vi "satellite simulator control.vi"() -> ()   [LabVIEW 2012]
uses:
  <vilib>/Utility/error.llb/DialogType.ctl
  <vilib>/DAQmx/create/channels.llb/DAQmx Create Channel (DO-Digital Output).vi
  <vilib>/Instr/_visa.llb/VISA Configure Serial Port (Instr).vi
  <vilib>/vision/NI_Vision_Development_Module.lvlib
  <vilib>/ptbypt/NI_PtbyPt.lvlib
panel:
  in  "Control Value":sgl=1.5 format="%.4f"
  in  "Control Mode":u16(ring) items=["Acceleration", "Speed", "Torque"]
  in  "Address":i32=11
  in  "Dst":i32=36
  in  "stop bits":u16(ring)=10 items=["1.0"=10, "1.5"=15, "2.0"=20]
  in  "VISA resource name (write) 2":refnum<visa-resource-name>="COM4"
  in  "flow control":u16(ring) items=["None"=0, "XON/XOFF"=1, "RTS/CTS"=2, "DTR/DSR"=4]
  in  "parity (0:none)":u16(ring) items=["None", "Odd", "Even", "Mark", "Space"]
  in  "data bits (8)":u16=8 min=5 max=8 step=1
  in  "baud rate (115200)":u32=115200
  out "bytes written":u32
  in  "bytes to read":u32=5
  out "read string":string
  out "bytes read":u32
  out "Filtered Ohmega":dbl format="%0.2f"
  in  "VISA resource name":refnum<visa-resource-name>
  out "read buffer":string
  out "Ohmega":dbl[](graph)
  out "Filtered Ohmega":dbl[](graph)
  in  "Floating":bool
  in  "Thruster 8":bool
  in  "Thruster 7":bool
  in  "Thruster 6":bool
  in  "Thruster 5":bool
  in  "Thruster 4":bool
  in  "Thruster 3":bool
  in  "Thruster 2":bool
  in  "Truster1":bool
  in  "Thrusters Bundled":bool=TRUE
  in  "Manual Control Mode (Default)":bool
  in  "Up":bool
  in  "Right":bool
  in  "Down":bool
  in  "Left":bool
  in  "Stop 2":bool
  in  "CntrClk":bool
  in  "ClkWise":bool
  in  "Angular Acceleration":u16(ring) items=["Fast", "Slow"]
  in  "Duty Cycle":dbl=1.0
  in  "Automatic PD Position Controller":bool
  in  "Pixel-Distance Ratio (pix/cm)":dbl=8.26
  in  "Remote Logger Status":bool
  in  "Downlink Object Data?":bool
  in  "Remote Port":u16=61557
  in  "Local Port":u16=61556
  in  "Remote Host":string="localhost"
  in  "broadcast":bool
  in  "Maintain Attitude":bool
  out "alpha":dbl
  out "Objects":T1(array[cluster]) {"Aspect Ratio" format="%.2f"; "Orientation" format="%.2f"; "Area" format="%.2f"; "Object Center"."Y" format="%.2f"; "Object Center"."X" format="%.2f"}
  in  "Y Center Correction":dbl
  in  "X Center Correction":dbl
  out "Offset Degree":dbl
  in  "Y Desired":dbl
  in  "X Desired":dbl
  out "Vx (cm/s)":dbl
  out "Vy (cm/s)":dbl
  in  "OK Button":bool
  in  "Air Floating Status":bool
  in  "Control Freq":u32=20
  in  "Alpha Desired":dbl
  in  "STOP":bool caption="stop (F)"
  out "Image Out":T2(plugin-control)
  out "alpha (deg)":dbl
  out "dx (cm)":dbl
  out "dy (cm)":dbl
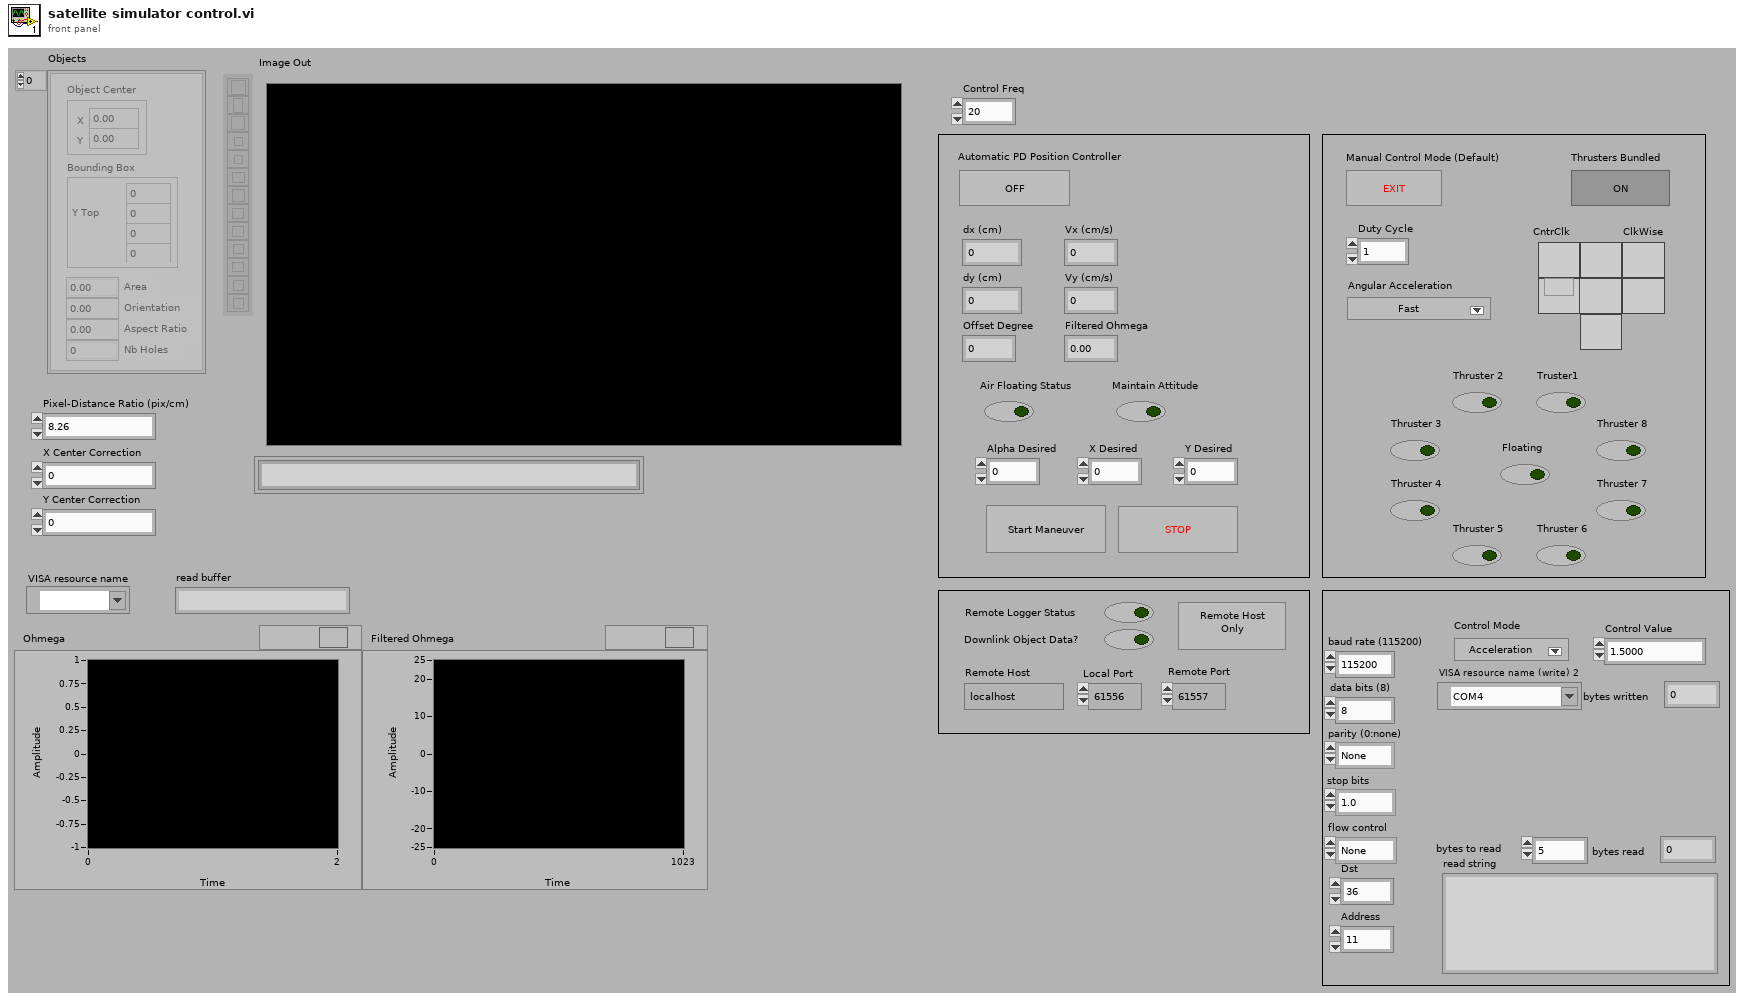
[diagram p1: front panel]
types:
  T1 = cluster{"Object Center":cluster{"X":sgl, "Y":sgl}, "Bounding Box":cluster{"X Left":i32, "Y Top":i32, "X Right":i32, "Y Bottom":i32}, "Area":sgl, "Orientation":sgl, "Aspect Ratio":sgl, "Nb Holes":i32}[]
  T2 = typedef "IMAQ Image.ctl" = refnum<image>
  T3 = typedef "DialogType.ctl" = u16
  T4 = cluster{"dx (cm)":dbl, "dy (cm)":dbl, "Offset Degree":dbl}
  T5 = cluster{"Objects":u16, "Threshold":i32, "Reject Border":bool, "Fill Holes":bool, "Min Object Size":bool, "Min Size":i32, "Max Object Size":bool, "Max Size":i32, "Show Search Area":bool, "Show Center":bool, "Show Bounding Box":bool}
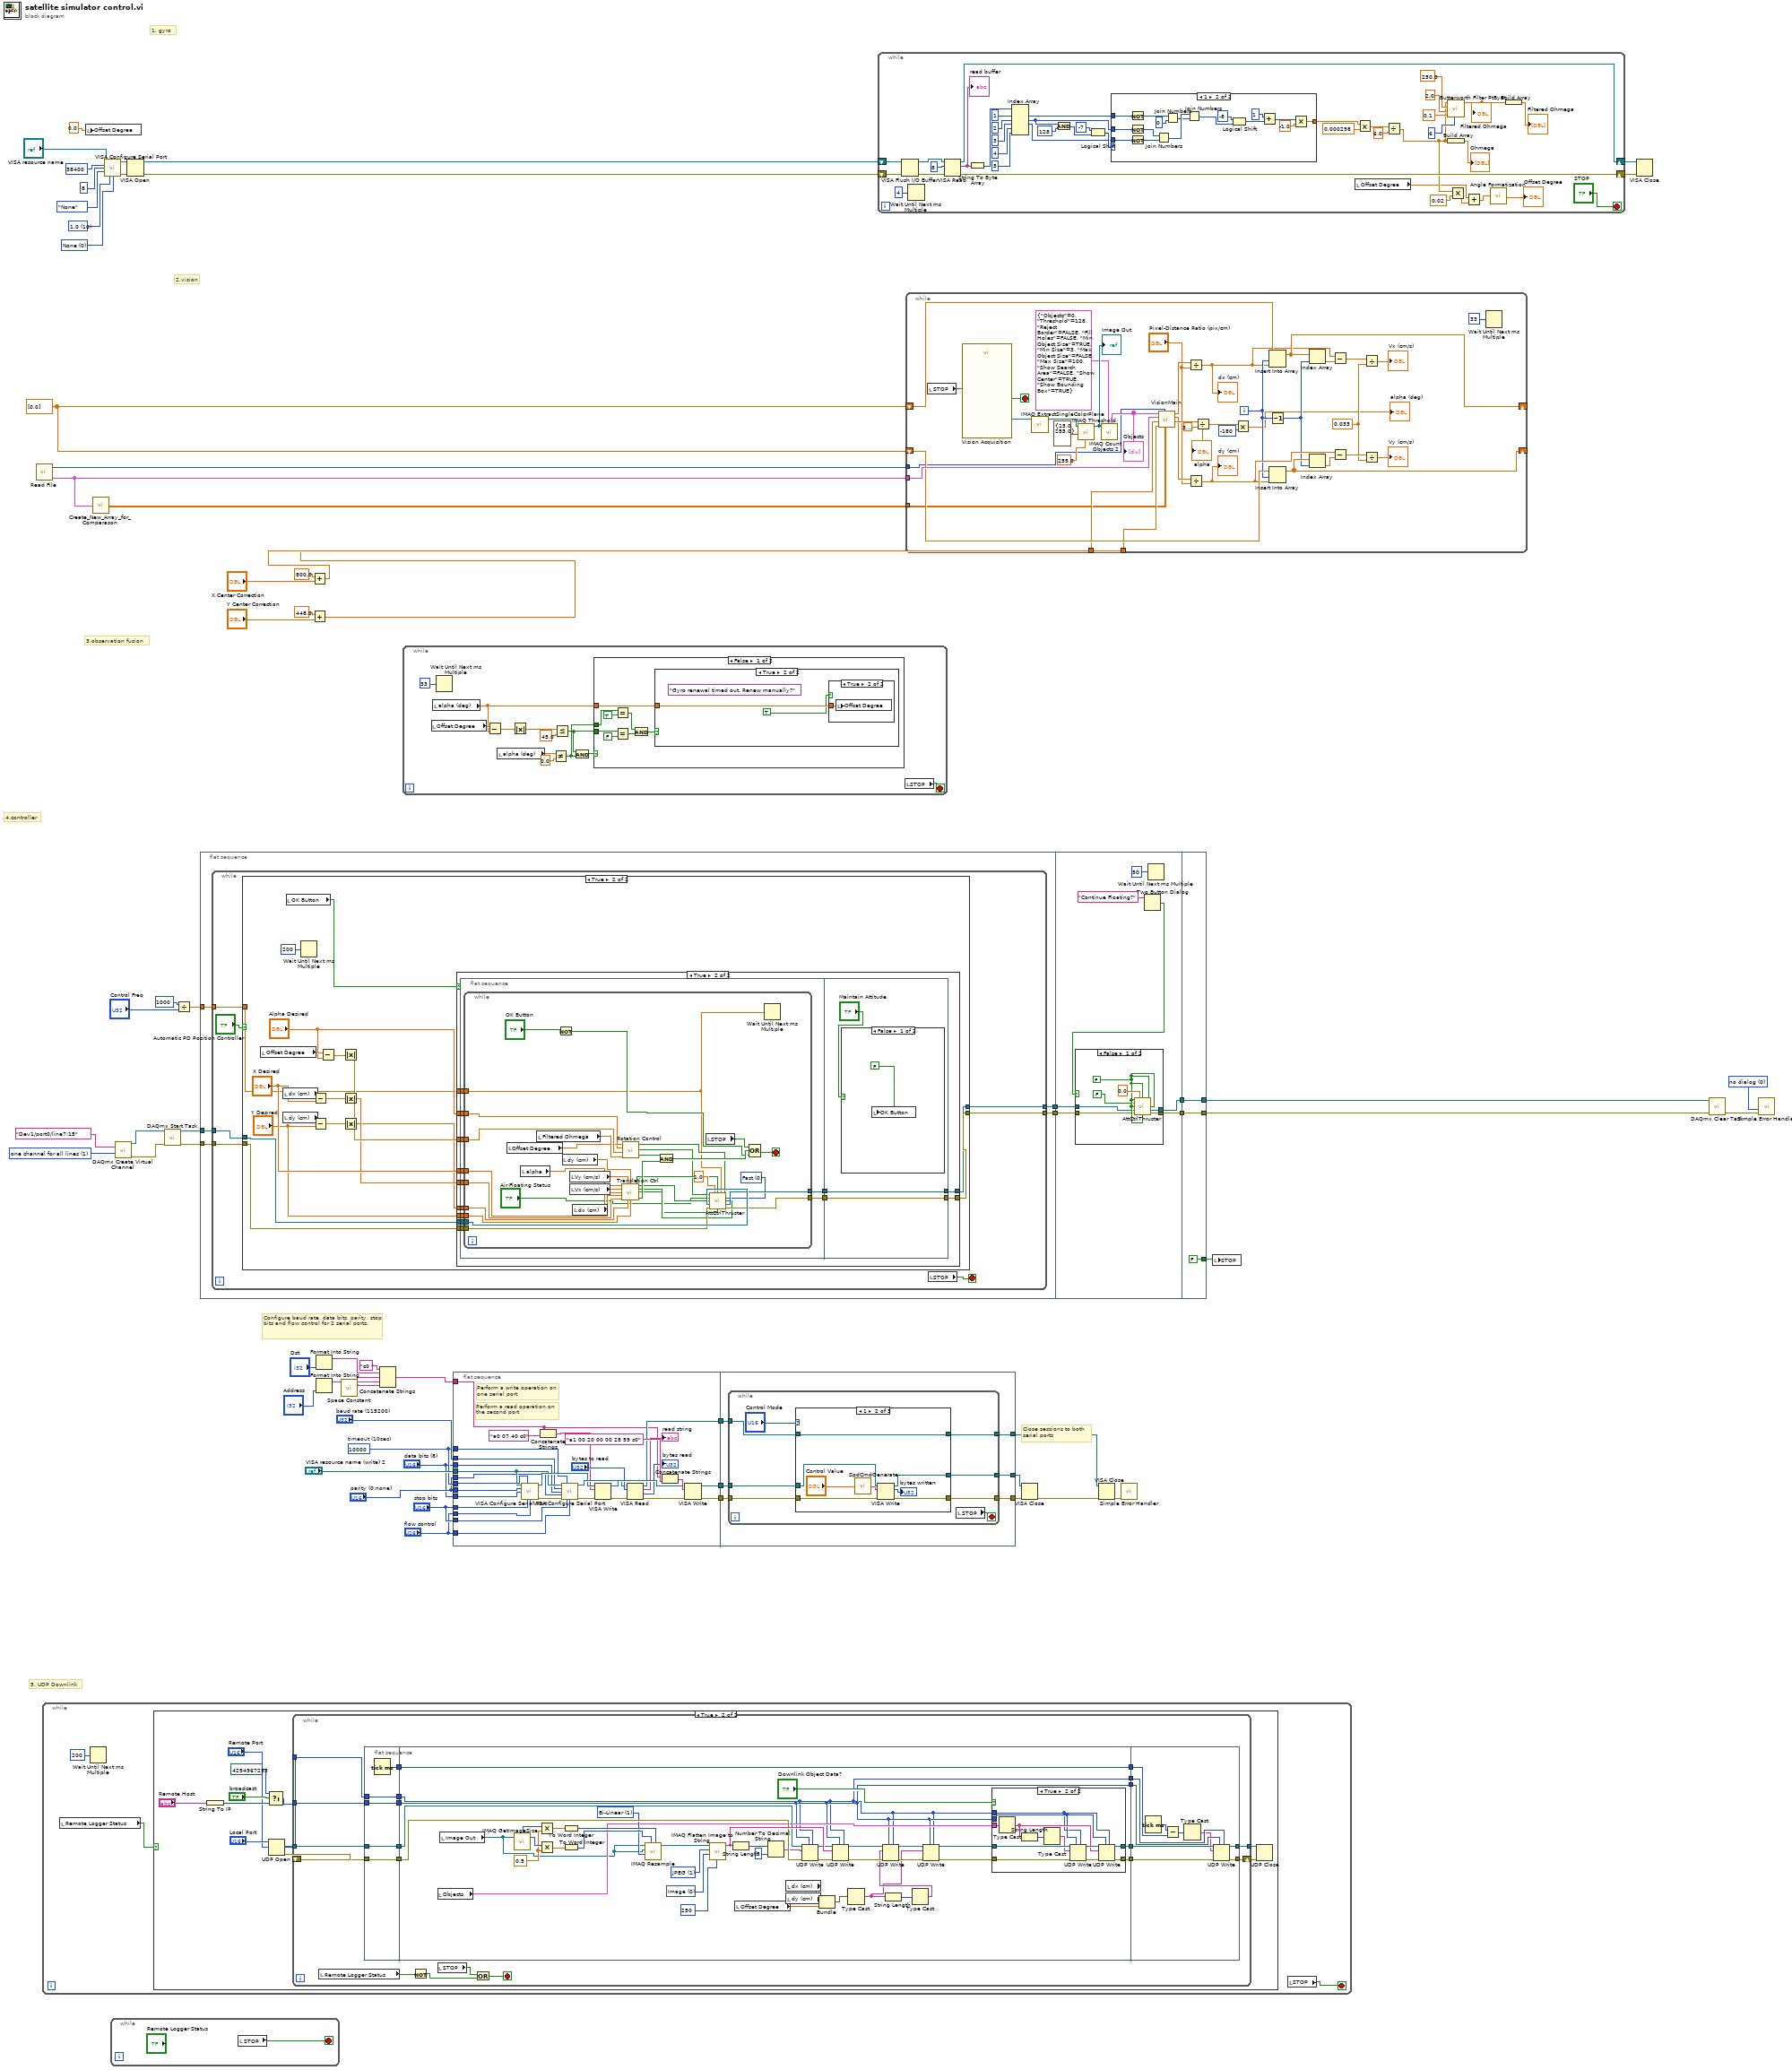
[diagram p0: block diagram]
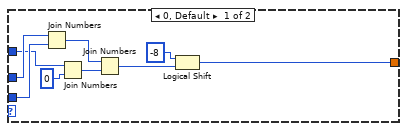
[diagram p4: hidden frame]
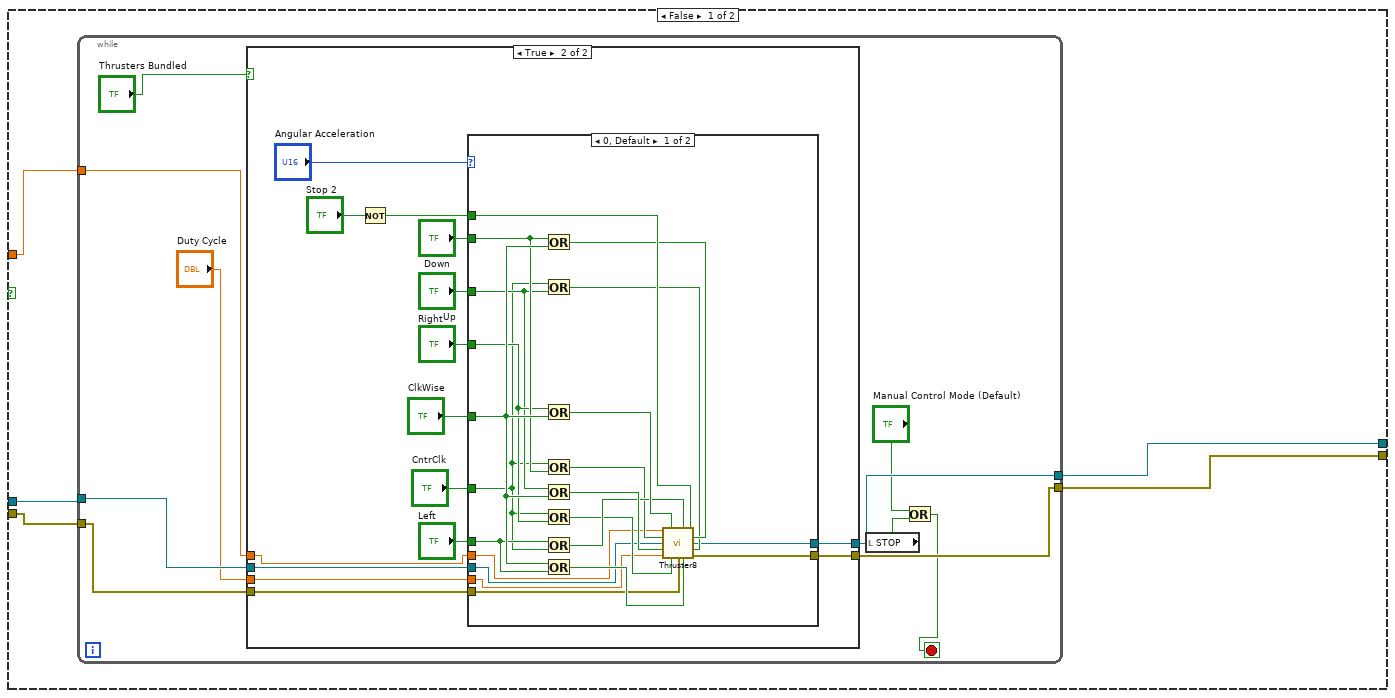
[diagram p7: hidden frame]
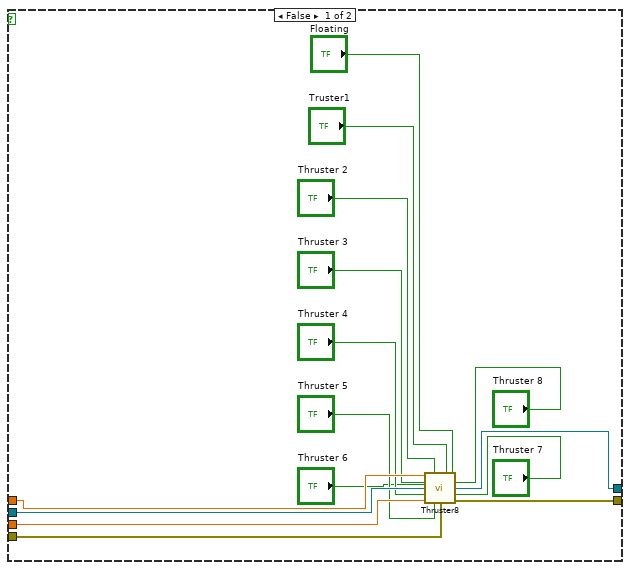
[diagram p8: hidden frame]
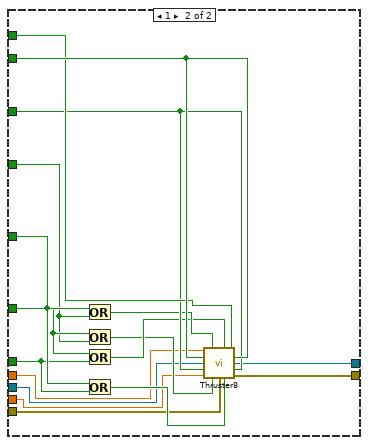
[diagram p9: hidden frame]
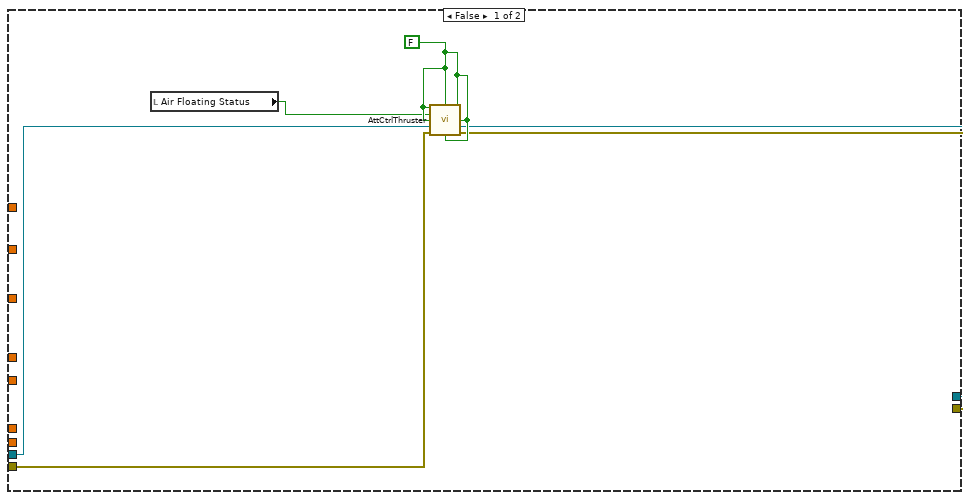
[diagram p10: hidden frame]
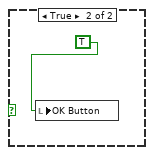
[diagram p11: hidden frame]
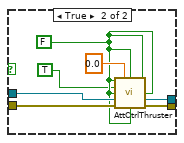
[diagram p12: hidden frame]
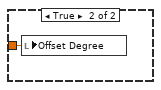
[diagram p15: hidden frame]
diagram:
  w6 = u32 10000  # timeout (10sec)
  w26 = u16 0 items=["None", "XON/XOFF", "RTS/CTS", "XON/XOFF & RTS/CTS", "DTR/DSR", "XON/XOFF & DTR/DSR"] ("flow control (0:none)")
  w28 = u16 10 items=["1.0"=10, "1.5"=15, "2.0"=20] ("stop bits (10: 1 bit)")
  w58 = T3 0 items=["no dialog", "OK message", "continue or stop message", "OK message + warnings", "continue/stop + warnings"] ("type of dialog (OK msg:1)")
  w61 = 1 items=["one channel for each line", "one channel for all lines"] ("line grouping")
  w47 = dbl[] [0.0]
  # "Close sessions to both serial ports"
  # "Configure baud rate, data bits, parity, stop bits and flow control for 2 serial ports."
  # "5. UDP Downlink"
  # "4.controller"
  # "3.observation fusion"
  # "2.vision"
  # "1. gyro"
  n1 = call "Read File.vi"() -> ("Objects"=w25:T1, "Total Obj"=w23:i32)  [unwired: 1 in]
  n2 = while {
    stop <- w65 stop-if-true
    n3 = local read "Remote Logger Status"() -> (w66:bool)
    n4 = Wait Until Next ms Multiple(millisecond multiple=u32 200) -> ()  [unwired: 1 out]
    n5 = case shown="True" w66 {
      frame False {
      }
      frame True {
        n6 = String To IP(1:"Remote Host") -> (0:w74:u32)
        n7 = Select(t=u32 4294967295, s="broadcast", f=w74) -> (s? t:f=w71:u32)
        n8 = UDP Open(11:"Local Port") -> (port=w70:refnum<k16>, 0:w69:errorcluster)  [unwired: 1 in, 4 out]
        n9 = while {
          tunnel: "Remote Port" -> [w97]
          tunnel: w71 -> [w96]
          tunnel: w70 -> [w95]
          tunnel: [w93] -> w68
          shift-right: [w92] -> w67
          shift-left: w69 -> [w94]
          stop <- w81 stop-if-true
          n10 = local read "Remote Logger Status"() -> (w79:bool)
          n11 = flat-sequence {
            tunnel: w95 -> [w99]
            tunnel: w97 -> [w100]
            tunnel: w96 -> [w101]
            tunnel: w94 -> [w102]
            tunnel: [w102] -> w91
            tunnel: [w101] -> w90
            tunnel: [w100] -> w89
            tunnel: [w99] -> w88
            tunnel: [w98] -> w87
            tunnel: [w122] -> w86
            tunnel: [w121] -> w85
            tunnel: w91 -> [w140]
            tunnel: w90 -> [w104]
            tunnel: w89 -> [w103]
            tunnel: w88 -> [w124]
            tunnel: [w123] -> w84
            tunnel: w87 -> [w123]
            tunnel: [w103] -> w83
            tunnel: [w104] -> w82
            tunnel: [w164] -> w93
            tunnel: [w158] -> w92
            tunnel: w86 -> [w159]
            tunnel: w85 -> [w165]
            tunnel: w84 -> [w166]
            tunnel: w83 -> [w163]
            tunnel: w82 -> [w162]
            frame #0 {
              n12 = Tick Count (ms)() -> (millisecond timer value=w98:u32)
            }
            frame #1 {
              w128 = u32 1 items=["Zero Order", "Bi-Linear", "Quadratic", "Cubic Spline"] ("Interpolation Type")
              w129 = 0.5
              w137 = 0 items=["Image", "Image and Vision Info", "Reference to Image"] ("Type of Flatten (Image and Vision Info)")
              w142 = 1 items=["None", "JPEG", "PACKED BINARY"] ("Compression (None)")
              n13 = local read "Objects"() -> (w119:T1)
              n14 = local read "Image Out"() -> (w118:T2)
              n15 = call "IMAQ GetImageSize"("Image"=w118) -> ("Y Resolution"=w130:i32, "X Resolution"=w131:i32)  [unwired: 3 in, 1 out]
              n16 = Multiply(x=w131, y=w129) -> (x*y=w133:dbl)
              n17 = Multiply(x=w130, y=w129) -> (x*y=w135:dbl)
              n18 = To Word Integer(number=w133) -> (16bit integer=w132:i16)
              n19 = To Word Integer(number=w135) -> (16bit integer=w134:i16)
              n20 = call "IMAQ Resample"("X Resolution"=w132, "Y Resolution"=w134, "Interpolation Type"=w128, "Image Dst"=w118, "Image Src"=w118) -> ("Image Dst Out"=w136:T2)  [unwired: 5 in, 1 out]
              n21 = call "IMAQ Flatten Image to String"("Quality (750)"=250, "Type of Flatten (Image and Vision Info)"=w137, "Compression (None)"=w142, "Image"=w136) -> ("Data String"=w141:string)  [unwired: 6 in, 1 out]
              n22 = String Length(string=w141) -> (length=w127:i32)
              n23 = local read "Offset Degree"() -> (w115:dbl)
              n24 = Number To Decimal String(number=w127, width (-)=i16 5) -> (decimal integer string=w126:string)
              n25 = local read "dx (cm)"() -> (w117:dbl)
              n26 = local read "dy (cm)"() -> (w116:dbl)
              n27 = UDP Write(address=w104, port or service name=w103, connection ID=w124, data in=w126, 8:w140) -> (error out=w139:errorcluster, 3:w138:refnum<k16>)  [unwired: 1 out]
              n28 = Bundle("dx (cm)"=w117, "dy (cm)"=w116, "Offset Degree"=w115) -> (w114:T4)  [unwired: 1 in]
              n29 = UDP Write(address=w104, port or service name=w103, connection ID=w138, data in=w141, 8:w139) -> (error out=w112:errorcluster, 3:w113:refnum<k16>)  [unwired: 1 out]
              n30 = Type Cast(x=w114) -> (*(type *) &x=w105:string)  [unwired: 1 in]
              n31 = String Length(string=w105) -> (length=w107:i32)
              n32 = Type Cast(x=w107) -> (*(type *) &x=w106:string)  [unwired: 1 in]
              n33 = UDP Write(address=w104, port or service name=w103, connection ID=w113, data in=w106, 8:w112) -> (error out=w111:errorcluster, 3:w109:refnum<k16>)  [unwired: 1 out]
              n34 = UDP Write(address=w104, port or service name=w103, connection ID=w109, data in=w105, 8:w111) -> (error out=w110:errorcluster, 3:w108:refnum<k16>)  [unwired: 1 out]
              n35 = case shown="True" "Downlink Object Data?" {
                tunnel: w119 -> [_ w157]
                tunnel: w110 -> [w145 w155]
                tunnel: [w145 w153] -> w122
                tunnel: w108 -> [w144 w152]
                tunnel: [w144 w150] -> w121
                tunnel: w104 -> [_ w147]
                tunnel: w103 -> [_ w146]
                frame False {
                }
                frame True {
                  n36 = Type Cast(x=w157) -> (*(type *) &x=w148:string)  [unwired: 1 in]
                  n37 = String Length(string=w148) -> (length=w156:i32)
                  n38 = Type Cast(x=w156) -> (*(type *) &x=w149:string)  [unwired: 1 in]
                  n39 = UDP Write(address=w147, port or service name=w146, connection ID=w152, data in=w149, 8:w155) -> (error out=w154:errorcluster, 3:w151:refnum<k16>)  [unwired: 1 out]
                  n40 = UDP Write(address=w147, port or service name=w146, connection ID=w151, data in=w148, 8:w154) -> (error out=w153:errorcluster, 3:w150:refnum<k16>)  [unwired: 1 out]
                }
              }
            }
            frame #2 {
              n41 = Tick Count (ms)() -> (millisecond timer value=w167:u32)
              n42 = Subtract(x=w167, y=w166) -> (x-y=w161:u32)
              n43 = Type Cast(x=w161) -> (*(type *) &x=w160:string)  [unwired: 1 in]
              n44 = UDP Write(address=w162, port or service name=w163, connection ID=w165, data in=w160, 8:w159) -> (error out=w158:errorcluster, 3:w164:refnum<k16>)  [unwired: 1 out]
            }
          }
          n45 = Not(x=w79) -> (.not. x?=w78:bool)
          n46 = local read "STOP"() -> (w80:bool)
          n47 = Or(x=w80, y=w78) -> (x .or. y?=w81:bool)
        }
        n48 = UDP Close(connection ID=w68, 8:w67) -> ()  [unwired: 2 out]
      }
    }
    n49 = local read "STOP"() -> (w65:bool)
  }
  n50 = local write "Offset Degree"(0.0 ("y")) -> ()
  n51 = call "Create_New_Array_for_Comparason.vi"("Captured Plots"=w25) -> ("Generated Distance Array"=w24:dbl[][])
  n52 = call-poly "VISA Configure Serial Port"("VISA resource name"="VISA resource name", "baud rate (9600)"=u32 38400, "data bits (8)"=u16 8, "parity (0:none)"=enum16{"None", "Odd", "Even", "Mark", "Space"}."None", "stop bits (10: 1 bit)"=w28, "flow control (0:none)"=w26) -> ("VISA resource name out"=w35:refnum<visa-resource-name>, "error out"=w34:errorcluster)  [unwired: 8 in]
  n53 = while {
    stop <- w168 stop-if-true
    n54 = local read "STOP"() -> (w168:bool)
  }
  n55 = call-poly <vilib>:"DAQmx Create Virtual Channel.vi"("lines"=tag "Dev1/port0/line7:15" ("Lines"), "line grouping"=w61) -> ("task out"=w59:refnum<k21>, "error out"=w60:errorcluster)  [unwired: 12 in]
  n56 = VISA Open(error in (no error)=w34, VISA resource name=w35) -> (VISA resource name=w33:refnum<visa-resource-name>, error out=w32:errorcluster)  [unwired: 3 in]
  n57 = call <vilib>:"DAQmx Start Task.vi"("task/channels in"=w59, "error in"=w60) -> ("task out"=w54:refnum<k21>, "error out"=w53:errorcluster)  [unwired: 12 in]
  n58 = Divide(x=u32 1000 ("milliseconds to wait"), y="Control Freq") -> (x/y=w50:dbl)
  n59 = flat-sequence {
    tunnel: w54 -> [w173]
    tunnel: w53 -> [w172]
    tunnel: w50 -> [w169]
    tunnel: [w171] -> w49
    tunnel: [w170] -> w48
    tunnel: w49 -> [w358]
    tunnel: w48 -> [w356]
    tunnel: [w357] -> w40
    tunnel: [w355] -> w39
    tunnel: [w374] -> w51
    tunnel: [w375] -> w52
    tunnel: w40 -> [w375]
    tunnel: w39 -> [w374]
    tunnel: [FALSE] -> w38
    frame #0 {
      n60 = while {
        tunnel: w173 -> [w180]
        tunnel: w172 -> [w179]
        tunnel: [w178] -> w171
        tunnel: [w177] -> w170
        tunnel: w169 -> [w175]
        stop <- w176 stop-if-true
        n61 = case shown="True" "Automatic PD Position Controller" {
          tunnel: w180 -> [w184 w282]
          tunnel: w179 -> [w183 w281]
          tunnel: [w181 w280] -> w178
          tunnel: [w182 w279] -> w177
          tunnel: w175 -> [w185 w265]
          frame False {
            n62 = while {
              tunnel: w185 -> [w195]
              tunnel: w184 -> [w194]
              tunnel: [w193] -> w182
              tunnel: [w192] -> w181
              tunnel: w183 -> [w191]
              stop <- w188 stop-if-true
              n63 = case shown="True" "Thrusters Bundled" {
                tunnel: w195 -> [w206 w218]
                tunnel: w194 -> [w210 w217]
                tunnel: [w207 w216] -> w193
                tunnel: [w208 w215] -> w192
                tunnel: w191 -> [w209 w214]
                tunnel: "Duty Cycle" -> [w205 w211]
                frame False {
                  n64 = call "Thruster8.vi"("period"=w206, "Thruster 2"="Thruster 2", "Truster1"="Truster1", "Floating"="Floating", "Thruster 3"="Thruster 3", "Thruster 8"="Thruster 8", "task in"=w210, "Thruster 4"="Thruster 4", "Thruster 7"="Thruster 7", "Duty Cycle"=w205, "Thruster 5"="Thruster 5", "error in"=w209, "Thruster 6"="Thruster 6") -> ("task out"=w207:refnum<k21>, "error out"=w208:errorcluster)  [unwired: 1 in]
                }
                frame True {
                  n65 = Not(x="Stop 2") -> (.not. x?=w212:bool)
                  n66 = case shown="0, Default" "Angular Acceleration" {
                    tunnel: w212 -> [w246 w262]
                    tunnel: "Down" -> [w238 w263]
                    tunnel: "Left" -> [w240 w256]
                    tunnel: "Up" -> [w234 w261]
                    tunnel: "Right" -> [w236 w254]
                    tunnel: "ClkWise" -> [w242 w260]
                    tunnel: "CntrClk" -> [w233 w257]
                    tunnel: w211 -> [w231 w252]
                    tunnel: w218 -> [w230 w251]
                    tunnel: w217 -> [w229 w247]
                    tunnel: [w228 w248] -> w216
                    tunnel: [w227 w249] -> w215
                    tunnel: w214 -> [w226 w250]
                    frame 0, Default {
                      n67 = Or(x=w238, y=w242) -> (x .or. y?=w241:bool)
                      n68 = Or(x=w233, y=w234) -> (x .or. y?=w232:bool)
                      n69 = Or(x=w236, y=w242) -> (x .or. y?=w244:bool)
                      n70 = Or(x=w233, y=w238) -> (x .or. y?=w237:bool)
                      n71 = Or(x=w234, y=w242) -> (x .or. y?=w245:bool)
                      n72 = Or(x=w233, y=w236) -> (x .or. y?=w235:bool)
                      n73 = Or(x=w240, y=w233) -> (x .or. y?=w239:bool)
                      n74 = Or(x=w242, y=w240) -> (x .or. y?=w243:bool)
                      n75 = call "Thruster8.vi"("period"=w230, "Thruster 2"=w244, "Truster1"=w239, "Floating"=w246, "Thruster 3"=w237, "Thruster 8"=w241, "task in"=w229, "Thruster 4"=w245, "Thruster 7"=w232, "Duty Cycle"=w231, "Thruster 5"=w235, "error in"=w226, "Thruster 6"=w243) -> ("task out"=w228:refnum<k21>, "error out"=w227:errorcluster)  [unwired: 1 in]
                    }
                    frame 1 {
                      n76 = Or(x=w260, y=w254) -> (x .or. y?=w259:bool)
                      n77 = Or(x=w257, y=w254) -> (x .or. y?=w253:bool)
                      n78 = Or(x=w257, y=w256) -> (x .or. y?=w255:bool)
                      n79 = Or(x=w260, y=w256) -> (x .or. y?=w258:bool)
                      n80 = call "Thruster8.vi"("period"=w251, "Thruster 2"=w259, "Truster1"=w255, "Floating"=w262, "Thruster 3"=w263, "Thruster 8"=w263, "task in"=w247, "Thruster 4"=w261, "Thruster 7"=w261, "Duty Cycle"=w252, "Thruster 5"=w253, "error in"=w250, "Thruster 6"=w258) -> ("task out"=w248:refnum<k21>, "error out"=w249:errorcluster)  [unwired: 1 in]
                    }
                  }
                }
              }
              n81 = local read "STOP"() -> (w190:bool)
              n82 = Or(x="Manual Control Mode (Default)", y=w190) -> (x .or. y?=w188:bool)
            }
          }
          frame True {
            n83 = local read "Offset Degree"() -> (w278:dbl)
            n84 = local read "dx (cm)"() -> (w274:dbl)
            n85 = local read "dy (cm)"() -> (w270:dbl)
            n86 = local read "OK Button"() -> (w266:bool)
            n87 = Wait Until Next ms Multiple(millisecond multiple=u32 200) -> ()  [unwired: 1 out]
            n88 = Subtract(x=w274, y="X Desired") -> (x-y=w272:dbl)
            n89 = Subtract(x=w270, y="Y Desired") -> (x-y=w268:dbl)
            n90 = Subtract(x=w278, y="Alpha Desired") -> (x-y=w276:dbl)
            n91 = Absolute Value(x=w276) -> (abs(x)=w275:dbl)
            n92 = Absolute Value(x=w272) -> (abs(x)=w271:dbl)
            n93 = Absolute Value(x=w268) -> (abs(x)=w267:dbl)
            n94 = case shown="True" w266 {
              tunnel: w282 -> [w286 w301]
              tunnel: w281 -> [w285 w300]
              tunnel: [w284 w299] -> w280
              tunnel: [w283 w298] -> w279
              tunnel: w265 -> [_ w297]
              tunnel: "Alpha Desired" -> [_ w296]
              tunnel: w275 -> [_ w295]
              tunnel: "X Desired" -> [_ w294]
              tunnel: w271 -> [_ w293]
              tunnel: "Y Desired" -> [_ w292]
              tunnel: w267 -> [_ w291]
              frame False {
                w288 = FALSE
                n95 = local read "Air Floating Status"() -> (w287:bool)
                n96 = call "AttCtrlThruster.vi"("ctclk"=w288, "Up"=w288, "clkwis"=w288, "Float"=w287, "Left"=w288, "Right"=w288, "task in"=w286, "error in"=w285, "Down"=w288) -> ("task out"=w283:refnum<k21>, "error out"=w284:errorcluster)  [unwired: 5 in]
              }
              frame True {
                n97 = flat-sequence {
                  tunnel: w301 -> [w312]
                  tunnel: w300 -> [w311]
                  tunnel: w297 -> [w308]
                  tunnel: w296 -> [w307]
                  tunnel: w295 -> [w306]
                  tunnel: w294 -> [w305]
                  tunnel: w293 -> [w304]
                  tunnel: w292 -> [w303]
                  tunnel: w291 -> [w302]
                  tunnel: [w310] -> w290
                  tunnel: [w309] -> w289
                  tunnel: [w348] -> w298
                  tunnel: [w349] -> w299
                  tunnel: w290 -> [w349]
                  tunnel: w289 -> [w348]
                  frame #0 {
                    n98 = while {
                      tunnel: w312 -> [w346]
                      tunnel: w311 -> [w345]
                      tunnel: [w343] -> w310
                      tunnel: [w344] -> w309
                      tunnel: w308 -> [w314]
                      tunnel: w307 -> [w324]
                      tunnel: w306 -> [w339]
                      tunnel: w305 -> [w323]
                      tunnel: w304 -> [w334]
                      tunnel: w303 -> [w322]
                      tunnel: w302 -> [w321]
                      stop <- w340 stop-if-true
                      w330 = u16 0 items=["Fast", "Slow"] ("Angular Acceleration")
                      n99 = local read "Offset Degree"() -> (w337:dbl)
                      n100 = local read "alpha"() -> (w318:dbl)
                      n101 = local read "Filtered Ohmega"() -> (w338:dbl)
                      n102 = Not(x="OK Button") -> (.not. x?=w319:bool)
                      n103 = local read "dy (cm)"() -> (w332:dbl)
                      n104 = local read "Vy (cm/s)"() -> (w333:dbl)
                      n105 = local read "Vx (cm/s)"() -> (w336:dbl)
                      n106 = local read "dx (cm)"() -> (w335:dbl)
                      n107 = call "Translation Ctrl.vi"("Alpha"=w318, "Filtered Speed Y"=w333, "Y In"=w332, "Filtered Speed X"=w336, "X In"=w335, "X Desired"=w323, "Original Difference X"=w334, "Original Difference Y"=w321, "Y Desired"=w322) -> ("Left"=w328:bool, "Right"=w327:bool, "Down"=w326:bool, "Up"=w325:bool, "Maneuver Complete?"=w329:bool)  [unwired: 2 in]
                      n108 = call "Rotation Control.vi"("Filtered Ohmega"=w338, "Original Difference"=w339, "Alpha Desired"=w324, "Alpha In"=w337) -> ("Maneuver Complete?"=w317:bool, "Counter-ClkWise Rot Ctrl"=w316:bool, "Clockwise Rot Ctrl"=w315:bool)
                      n109 = And(x=w317, y=w329) -> (x .and. y?=w331:bool)
                      n110 = local read "STOP"() -> (w341:bool)
                      n111 = call "AttCtrlThruster.vi"("ctclk"=w316, "Duty Cycle"=1.0, "Up"=w325, "Period"=w314, "clkwis"=w315, "Float"="Air Floating Status", "Angular Acceleration"=w330, "Left"=w328, "Right"=w327, "task in"=w346, "error in"=w345, "Down"=w326) -> ("task out"=w344:refnum<k21>, "error out"=w343:errorcluster)  [unwired: 2 in]
                      n112 = Compound Arithmetic op=OR(w341, w331, w319) -> (w340:bool)
                      n113 = Wait Until Next ms Multiple(millisecond multiple=w314) -> ()  [unwired: 1 out]
                    }
                  }
                  frame #1 {
                    n114 = case shown="False" "Maintain Attitude" {
                      frame False {
                        n115 = local write "OK Button"(FALSE) -> ()
                      }
                      frame True {
                        n116 = local write "OK Button"(TRUE) -> ()
                      }
                    }
                  }
                }
              }
            }
          }
        }
        n117 = local read "STOP"() -> (w176:bool)
      }
    }
    frame #1 {
      n118 = Two Button Dialog(message="Continue Floating?") -> (T button?=w352:bool)  [unwired: 2 in]
      n119 = case shown="False" w352 {
        tunnel: w358 -> [w361 w372]
        tunnel: [w359 w371] -> w357
        tunnel: w356 -> [w362 w370]
        tunnel: [w360 w369] -> w355
        frame False {
          w364 = FALSE
          n120 = call "AttCtrlThruster.vi"("ctclk"=w364, "Duty Cycle"=0.0, "Up"=w364, "clkwis"=w364, "Float"=FALSE, "Left"=w364, "Right"=w364, "task in"=w362, "error in"=w361, "Down"=w364) -> ("task out"=w360:refnum<k21>, "error out"=w359:errorcluster)  [unwired: 4 in]
        }
        frame True {
          w367 = FALSE
          n121 = call "AttCtrlThruster.vi"("ctclk"=w367, "Duty Cycle"=0.0, "Up"=w367, "clkwis"=w367, "Float"=TRUE, "Left"=w367, "Right"=w367, "task in"=w370, "error in"=w372, "Down"=w367) -> ("task out"=w369:refnum<k21>, "error out"=w371:errorcluster)  [unwired: 4 in]
        }
      }
      n122 = Wait Until Next ms Multiple(millisecond multiple=u32 50) -> ()  [unwired: 1 out]
    }
    frame #2 {
    }
  }
  n123 = Add(x=800.0 ("c_x"), y="X Center Correction") -> (x+y=w44:dbl)
  n124 = Add(x=448.0 ("c_y"), y="Y Center Correction") -> (x+y=w41:dbl)
  n125 = Format Into String("Dst") -> (resulting string=w13:string)  [unwired: 3 in, 1 out]
  n126 = Format Into String("Address") -> (resulting string=w15:string)  [unwired: 3 in, 1 out]
  n127 = call <vilib>:"Space Constant.vi"() -> ("String"=w12:string)
  n128 = Concatenate Strings("c0 " ("string"), w13, w12, w15, w12) -> (w1:string)
  n129 = while {
    stop <- w386 stop-if-true
    n130 = local read "Offset Degree"() -> (w385:dbl)
    n131 = local read "alpha (deg)"() -> (w381:dbl)
    n132 = Wait Until Next ms Multiple(millisecond multiple=u32 33) -> ()  [unwired: 1 out]
    n133 = Subtract(x=w385, y=w381) -> (x-y=w384:dbl)
    n134 = local read "alpha (deg)"() -> (w379:dbl)
    n135 = Absolute Value(x=w384) -> (abs(x)=w383:dbl)
    n136 = Not Equal?(x=w379, y=0.0) -> (x != y?=w377:bool)
    n137 = Less Or Equal?(x=w383, y=45.0) -> (x <= y?=w376:bool)
    n138 = And(x=w376, y=w377) -> (x .and. y?=w380:bool)
    n139 = case shown="False" w380 {
      tunnel: w381 -> [w388 w399]
      tunnel: w377 -> [w390 _]
      tunnel: w376 -> [w389 _]
      frame False {
        n140 = Equal?(x=w390, y=TRUE) -> (x = y?=w394:bool)
        n141 = Equal?(x=w389, y=FALSE) -> (x = y?=w393:bool)
        n142 = And(x=w394, y=w393) -> (x .and. y?=w391:bool)
        n143 = case shown="True" w391 {
          tunnel: w388 -> [_ w397]
          frame False {
          }
          frame True {
            (unwired) "Gyro renewal timed out. Renew manually?" ("message")
            n144 = case shown="True" TRUE {
              tunnel: w397 -> [_ w398]
              frame False {
              }
              frame True {
                n145 = local write "Offset Degree"(w398) -> ()
              }
            }
          }
        }
      }
      frame True {
        n146 = local write "Offset Degree"(w399) -> ()
      }
    }
    n147 = local read "STOP"() -> (w386:bool)
  }
  n148 = flat-sequence {
    tunnel: [w403] -> w11
    tunnel: [w417] -> w10
    tunnel: [w416] -> w9
    tunnel: w6 -> [w415]
    tunnel: "VISA resource name (write) 2" -> [w414]
    tunnel: "stop bits" -> [w413]
    tunnel: "flow control" -> [w412]
    tunnel: "baud rate (115200)" -> [w411]
    tunnel: "data bits (8)" -> [w410]
    tunnel: "parity (0:none)" -> [w409]
    tunnel: w6 -> [w408]
    tunnel: "parity (0:none)" -> [w407]
    tunnel: "data bits (8)" -> [w406]
    tunnel: "stop bits" -> [w405]
    tunnel: "flow control" -> [w404]
    tunnel: w1 -> [w400]
    tunnel: [w434] -> w20
    tunnel: [w432] -> w19
    tunnel: [w430] -> w18
    tunnel: w11 -> [w435]
    tunnel: w10 -> [w433]
    tunnel: w9 -> [w431]
    frame #0 {
      # "Perform a write operation on one serial port"
      # "Perform a read operation on the second port"
      n149 = call-poly "VISA Configure Serial Port"("VISA resource name"=w414, "timeout (10sec)"=w415, "baud rate (9600)"=w407, "data bits (8)"=w406, "stop bits (10: 1 bit)"=w413, "flow control (0:none)"=w412) -> ("VISA resource name out"=w418:refnum<visa-resource-name>, "error out"=w423:errorcluster)  [unwired: 3 in, 5 out]
      n150 = Concatenate Strings(w400, "a0 07 40 c0" ("string")) -> (w401:string)
      n151 = call-poly "VISA Configure Serial Port"("VISA resource name"=w414, "timeout (10sec)"=w408, "baud rate (9600)"=w411, "data bits (8)"=w410, "parity (0:none)"=w409, "error in (no error)"=w423, "stop bits (10: 1 bit)"=w405, "flow control (0:none)"=w404) -> ("VISA resource name out"=w419:refnum<visa-resource-name>, "error out"=w424:errorcluster)  [unwired: 2 in, 4 out]
      n152 = VISA Write(VISA resource name=w418, write buffer=w401, error in (no error)=w424) -> (VISA resource name out=w426:refnum<visa-resource-name>, error out=w425:errorcluster)  [unwired: 1 out]
      n153 = VISA Read(VISA resource name=w419, byte count="bytes to read", error in (no error)=w425) -> (VISA resource name out=w403:refnum<visa-resource-name>, read buffer=→"read string":string, return count=→"bytes read":u32, error out=w427:errorcluster)
      n154 = Concatenate Strings(w400, "a1 00 20 00 00 28 59 c0" ("string")) -> (w429:string)
      n155 = VISA Write(VISA resource name=w426, write buffer=w429, error in (no error)=w427) -> (VISA resource name out=w417:refnum<visa-resource-name>, error out=w416:errorcluster)  [unwired: 1 out]
    }
    frame #1 {
      n156 = while {
        tunnel: w435 -> [w443]
        tunnel: [w442] -> w434
        tunnel: w433 -> [w441]
        tunnel: [w440] -> w432
        tunnel: w431 -> [w439]
        tunnel: [w438] -> w430
        stop <- w437 stop-if-true
        n157 = case shown="1" "Control Mode" {
          tunnel: w443 -> [_ w444 _]
          tunnel: [_ w444 _] -> w442
          tunnel: w441 -> [_ w451 _]
          tunnel: [_ w450 _] -> w440
          tunnel: w439 -> [_ w449 _]
          tunnel: [_ w448 _] -> w438
          frame 0, Default {
          }
          frame 1 {
            n158 = call "SpdCmdGenerate.vi"("Speed"="Control Value") -> ("CMD code"=w446:string)
            n159 = VISA Write(VISA resource name=w451, write buffer=w446, error in (no error)=w449) -> (VISA resource name out=w450:refnum<visa-resource-name>, return count=→"bytes written":u32, error out=w448:errorcluster)
          }
          frame 2 {
          }
        }
        n160 = local read "STOP"() -> (w437:bool)
      }
    }
  }
  n161 = while {
    shift-right: [w459] -> w30
    shift-left: w32 -> [w489]
    shift-right: [w460] -> w31
    shift-left: w33 -> [w490]
    stop <- "STOP" stop-if-true
    n162 = VISA Flush I/O Buffer(VISA resource name=w490, error in (no error)=w489) -> (VISA resource name out=w488:refnum<visa-resource-name>, error out=w487:errorcluster)  [unwired: 1 in]
    n163 = Wait Until Next ms Multiple(millisecond multiple=u32 4) -> ()  [unwired: 1 out]
    n164 = VISA Read(VISA resource name=w488, byte count=u32 8, error in (no error)=w487) -> (VISA resource name out=w460:refnum<visa-resource-name>, read buffer=w461:string, error out=w459:errorcluster)  [unwired: 1 out]
    "read buffer" <- w461
    n165 = String To Byte Array(string=w461) -> (unsigned byte array=w482:u8[])
    n166 = Index Array(array=w482, index #1=1 ("index"), index #2=2 ("index"), index #3=3 ("index"), index #4=4 ("index"), index #5=5 ("index")) -> (element #1=w466:u8, element #2=w465:u8, element #3=w464:u8)  [unwired: 2 out]
    n167 = And(x=w465, y=u8 128) -> (x .and. y?=w476:u8)
    n168 = Logical Shift(y=i16 -7, x=w476) -> (x << y=w474:u8)
    n169 = case shown="1" w474 {
      tunnel: [w492 w501] -> w478
      tunnel: w466 -> [w493 w511]
      tunnel: w465 -> [w495 w510]
      tunnel: w464 -> [w494 w509]
      frame 0, Default {
        n170 = Join Numbers(hi=w495, lo=w494) -> ((hi.lo)=w500:u16)
        n171 = Join Numbers(hi=w493, lo=u8 0) -> ((hi.lo)=w498:u16)
        n172 = Join Numbers(hi=w500, lo=w498) -> ((hi.lo)=w497:u32)
        n173 = Logical Shift(y=i16 -8, x=w497) -> (x << y=w492:u32)
      }
      frame 1 {
        n174 = Not(x=w511) -> (.not. x?=w506:u8)
        n175 = Not(x=w510) -> (.not. x?=w508:u8)
        n176 = Not(x=w509) -> (.not. x?=w507:u8)
        n177 = Join Numbers(hi=w508, lo=w507) -> ((hi.lo)=w516:u16)
        n178 = Join Numbers(hi=w506, lo=u8 0) -> ((hi.lo)=w514:u16)
        n179 = Join Numbers(hi=w516, lo=w514) -> ((hi.lo)=w513:u32)
        n180 = Logical Shift(y=i16 -8, x=w513) -> (x << y=w505:u32)
        n181 = Add(x=u32 1, y=w505) -> (x+y=w502:u32)
        n182 = Multiply(x=w502, y=-1.0) -> (x*y=w501:dbl)
      }
    }
    n183 = local read "Offset Degree"() -> (w455:dbl)
    n184 = Multiply(x=w478, y=0.000298) -> (x*y=w484:dbl)
    n185 = Divide(x=w484, y=6.0) -> (x/y=w456:dbl)
    n186 = call <vilib>:"Butterworth Filter PtByPt.vi"("order"=6, "low cutoff freq: fl"=0.1, "high cutoff freq: fh"=2.0, "sampling freq: fs"=250.0, "x"=w456) -> ("Filtered x"=w468:dbl)  [unwired: 4 in, 1 out]
    "Filtered Ohmega" <- w468
    n187 = Build Array(w456) -> (→"Ohmega":dbl[])
    n188 = Multiply(x=w456, y=0.02) -> (x*y=w454:dbl)
    n189 = Add(x=w455, y=w454) -> (x+y=w453:dbl)
    n190 = call "Angle Formatization.vi"("Alpha"=w453) -> ("Alpha Formatized"=→"Offset Degree":dbl)
    n191 = Build Array(w468) -> (→"Filtered Ohmega":dbl[])
  }
  n192 = while {
    tunnel: w25 -> [w543]
    shift-right: [w540] -> _
    shift-left: w47 -> [w541]
    shift-right: [w529] -> _
    shift-left: w47 -> [w532]
    tunnel: w41 -> [w522]
    tunnel: w44 -> [w521]
    tunnel: w24 -> [w518]
    tunnel: w23 -> [w517]
    i -> [w531]
    stop <- w554 stop-if-true
    w525 = 0.033 ("y")
    n193 = local read "STOP"() -> (w545:bool)
    n194 = call "Vision Acquisition"("Stop (F)"=w545) -> ("Image Out"=w549:T2, "Stopped"=w554:bool)  [unwired: 24 in, 1 out]
    n195 = call "IMAQ ExtractSingleColorPlane"("Image Src"=w549) -> ("Image Dst Out"=w553:T2)  [unwired: 9 in, 1 out]
    n196 = call "IMAQ Threshold"("Replace Value"=sgl 255.0 ("replace value"), "Range"=cluster{"lower value":sgl, "upper value":sgl} {"lower value"=15.0, "upper value"=255.0} ("threshold"), "Image Src"=w553) -> ("Image Dst Out"=w550:T2)  [unwired: 7 in, 1 out]
    "Image Out" <- w550
    n197 = call "IMAQ Count Objects 2"("Settings"=T5 {"Objects"=0, "Threshold"=128, "Reject Border"=FALSE, "Fill Holes"=FALSE, "Min Object Size"=TRUE, "Min Size"=3, "Max Object Size"=FALSE, "Max Size"=100, "Show Search Area"=FALSE, "Show Center"=TRUE, "Show Bounding Box"=TRUE}, "Image"=w550) -> ("Objects"=w544:T1)  [unwired: 5 in, 4 out]
    "Objects" <- w544
    n198 = call "VisionMain.vi"("Generated Distance Array"=w518, "Database Total Points"=w517, "Y Center"=w522, "X Center"=w521, "Original Plots"=w543, "Plots Captured"=w544) -> ("alpha"=w542:dbl, "dy"=w538:dbl, "dx"=w533:dbl)  [unwired: 3 in]
    "alpha" <- w542
    n199 = Divide(x=w533, y="Pixel-Distance Ratio (pix/cm)") -> (x/y=w528:dbl)
    "dx (cm)" <- w528
    n200 = Divide(x=w538, y="Pixel-Distance Ratio (pix/cm)") -> (x/y=w537:dbl)
    "dy (cm)" <- w537
    n201 = Divide(x=w542, y=3.141592653589793) -> (x/y=w547:dbl)
    n202 = Multiply(x=w547, y=-180) -> (x*y=→"alpha (deg)":dbl)
    n203 = Insert Into Array(array=w532, index=w531, new element=w528) -> (w529:dbl[])
    n204 = Insert Into Array(array=w541, index=w531, new element=w537) -> (w540:dbl[])
    n205 = Decrement(x=w531) -> (x-1=w530:i32)
    n206 = Index Array(array=w529, index=w530) -> (element=w527:dbl)
    n207 = Index Array(array=w540, index=w530) -> (element=w539:dbl)
    n208 = Subtract(x=w528, y=w527) -> (x-y=w526:dbl)
    n209 = Subtract(x=w537, y=w539) -> (x-y=w536:dbl)
    n210 = Divide(x=w526, y=w525) -> (x/y=→"Vx (cm/s)":dbl)
    n211 = Divide(x=w536, y=w525) -> (x/y=→"Vy (cm/s)":dbl)
    n212 = Wait Until Next ms Multiple(millisecond multiple=u32 33) -> ()  [unwired: 1 out]
  }
  n213 = VISA Close(VISA resource name=w19, error in (no error)=w18) -> (error out=w22:errorcluster)
  n214 = VISA Close(VISA resource name=w20, error in (no error)=w22) -> (error out=w21:errorcluster)
  n215 = call <vilib>:"Simple Error Handler.vi"("error in (no error)"=w21) -> ()  [unwired: 1 in, 8 out]
  n216 = local write "STOP"(w38) -> ()
  n217 = VISA Close(VISA resource name=w31, error in (no error)=w30) -> ()  [unwired: 1 out]
  n218 = call <vilib>:"DAQmx Clear Task.vi"("task in"=w51, "error in"=w52) -> ("error out"=w57:errorcluster)  [unwired: 13 in]
  n219 = call <vilib>:"Simple Error Handler.vi"("type of dialog (OK msg:1)"=w58, "error in (no error)"=w57) -> ()  [unwired: 3 in, 5 out]
